vi "create_folder_SD.vi"(2 "base path":path, 3 "Name":string, 4 "error in":errorcluster) -> (0 "appended path":path, 1 "error out":errorcluster)   [LabVIEW 2015]
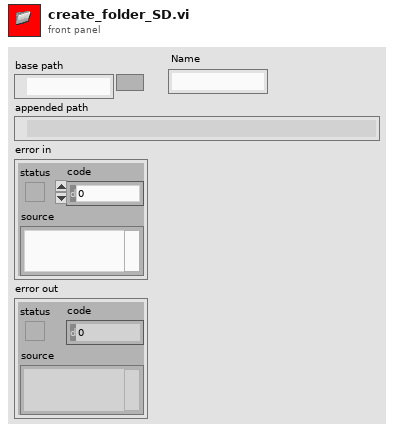
[diagram p1: front panel]
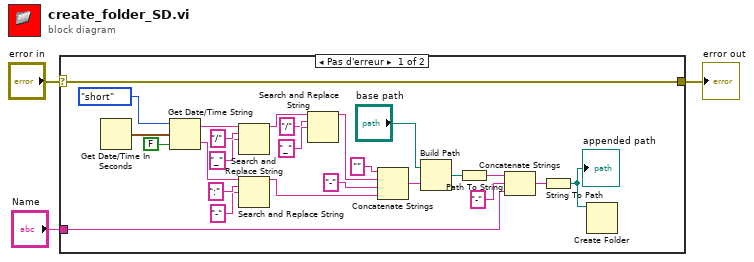
[diagram p0: block diagram]
diagram:
  n1 = case shown="Pas d'erreur" "error in" {
    selector: "error in" -> [w28 w29]
    tunnel: [w28 w29] -> w2
    tunnel: "Name" -> [w4 _]
    frame No Error {
      n2 = Get Date/Time In Seconds() -> (seconds since 1Jan1904=w25:timestamp)
      n3 = Get Date/Time String(date format (0)=enum16{"short", "long", "abbreviated"}."short", seconds (now)=w25, want seconds? (F)=FALSE) -> (date string=w16:string, time string=w20:string)
      n4 = Search and Replace String(input string=w16, search string="/", replace string="_" ("replace string (\"\")")) -> (result string=w11:string)  [unwired: 5 in, 3 out]
      n5 = Search and Replace String(input string=w20, search string=":", replace string="-" ("replace string (\"\")")) -> (result string=w19:string)  [unwired: 5 in, 3 out]
      n6 = Search and Replace String(input string=w11, search string="/", replace string="_" ("replace string (\"\")")) -> (result string=w10:string)  [unwired: 5 in, 3 out]
      n7 = Concatenate Strings("" ("name or relative path"), w10, "-" ("string"), w19) -> (w24:string)
      n8 = Build Path(base path="base path", name or relative path=w24) -> (appended path=w5:path)
      n9 = Path To String(path=w5) -> (string=w7:string)
      n10 = Concatenate Strings(w7, "-" ("string"), w4) -> (w9:string)
      n11 = String To Path(string=w9) -> (path=w6:path)
      "appended path" <- w6
      n12 = Create Folder(path (use dialog)=w6) -> ()  [unwired: 2 in, 3 out]
    }
    frame Error {
    }
  }
  "error out" <- w2
